vi "SplitConfig.vi"(8 "error in (no error)":errorcluster, 10 "Config":string, 11 "FileReader in":refnum<class "FileReader.lvclass">) -> (0 "error out":errorcluster, 1 "Range":string, 2 "triggering":string, 3 "FileReader out":refnum<class "FileReader.lvclass">, 4 "limits":string)   [LabVIEW 2011, in "Tools.lvlib" / "Filing.lvlib" / "FileReader.lvclass"]
uses:
  FileReader.lvclass
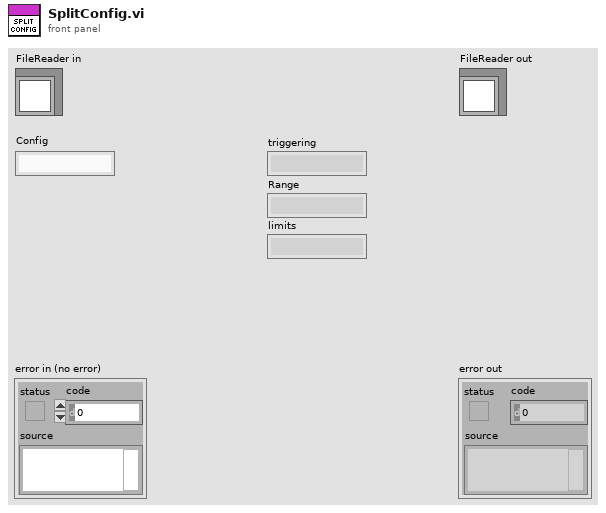
[diagram p1: front panel]
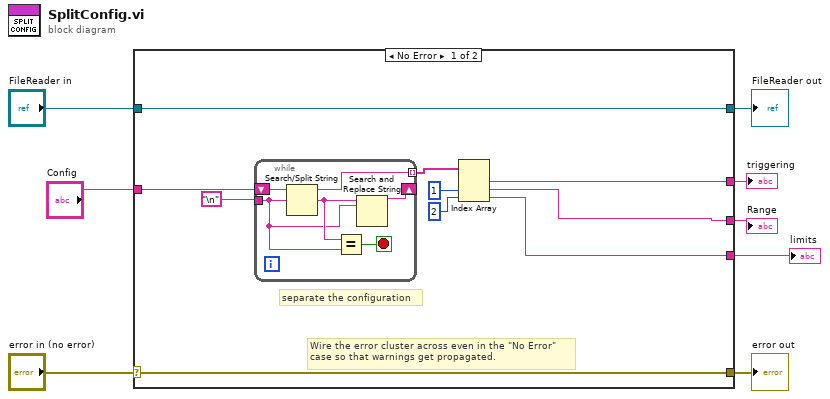
[diagram p0: block diagram]
diagram:
  n1 = case shown="No Error" "error in (no error)" {
    selector: "error in (no error)" -> [w17 w26]
    tunnel: [w17 w26] -> w7
    tunnel: [w18 w25] -> w5
    tunnel: "FileReader in" -> [w18 w25]
    tunnel: "Config" -> [w13 _]
    tunnel: [w11 _] -> w3
    tunnel: [w10 _] -> w2
    tunnel: [w9 _] -> w1
    frame No Error {
      # "separate the configuration"
      # "Wire the error cluster across even in the \"No Error\"\ncase so that warnings get propagated."
      n2 = while {
        tunnel: "\n" -> [w19]
        shift-right: [w20] -> _
        shift-left: w13 -> [w24]
        tunnel: [w23] -> w15 mode=indexing
        stop <- w22 stop-if-true
        n3 = Search/Split String(string=w24, search string/char (-)=w19) -> (substring before match=w23:string, match + rest of string=w21:string)  [unwired: 1 in, 1 out]
        n4 = Equal?(x=w21, y=w19) -> (x = y?=w22:bool)
        n5 = Search and Replace String(input string=w21, search string=w19) -> (result string=w20:string)  [unwired: 6 in, 3 out]
      }
      n6 = Index Array(array=w15, index #2=1, index #3=2) -> (element #1=w11:string, element #2=w10:string, element #3=w9:string)  [unwired: 1 in]
    }
    frame Error {
    }
  }
  "error out" <- w7
  "FileReader out" <- w5
  "triggering" <- w3
  "Range" <- w2
  "limits" <- w1
